vi "Get Axis Motion Status Motor Modified.vi"(8 "error in (no error)":errorcluster, 9 "Axis (1)":i32=1 min=1 max=3, 10 "VISA resource name":refnum<visa-resource-name>, 11 "ESP301 in":refnum<class "ESP301.lvclass">) -> (0 "error out":errorcluster, 1 "Motion Done":bool, 2 "VISA resource name out":refnum<visa-resource-name>, 3 "ESP301 out":refnum<class "ESP301.lvclass">)   [LabVIEW 2020, in "ESP301.lvclass"]
uses:
  ESP301.lvclass
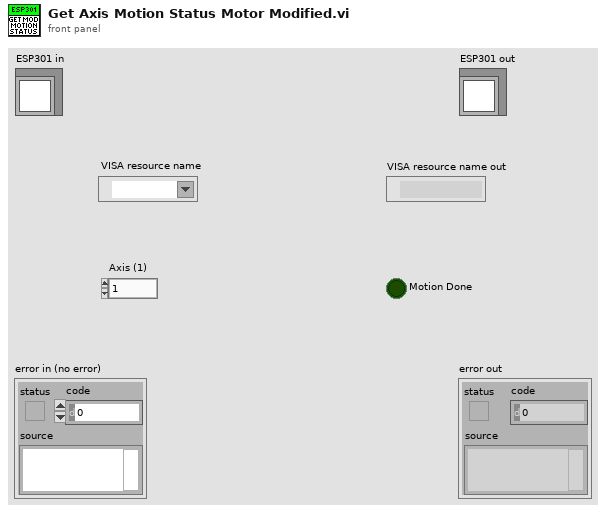
[diagram p1: front panel]
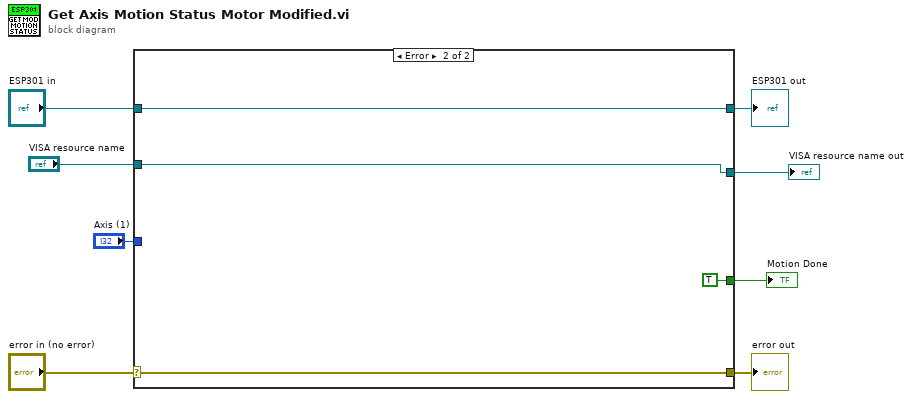
[diagram p0: block diagram]
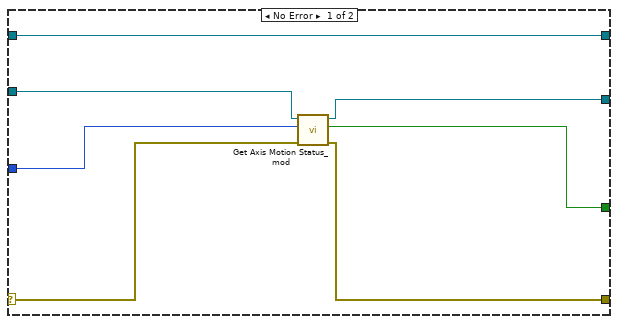
[diagram p2: hidden frame]
diagram:
  n1 = case shown="Error" "error in (no error)" {
    selector: "error in (no error)" -> [w13 w19]
    tunnel: [w12 w19] -> w7
    tunnel: [w15 w18] -> w5
    tunnel: "ESP301 in" -> [w15 w18]
    tunnel: "VISA resource name" -> [w14 w16]
    tunnel: "Axis (1)" -> [w11 _]
    tunnel: [w10 w16] -> w2
    tunnel: [w9 TRUE ("Motion Done")] -> w1
    frame No Error {
      n2 = call "Get Axis Motion Status_mod.vi"("error in (no error)"=w13, "Axis (1)"=w11, "VISA resource name"=w14) -> ("error out"=w12:errorcluster, "Motion Done"=w9:bool, "VISA resource name out"=w10:refnum<visa-resource-name>)  [unwired: 2 in]
    }
    frame Error {
    }
  }
  "error out" <- w7
  "ESP301 out" <- w5
  "VISA resource name out" <- w2
  "Motion Done" <- w1
